vi "ziModGetSweeperHeader.vi"(8 "Error In":errorcluster, 10 "ModResults":T2, 11 "ModHandle In":T5 {"ModHandle" format="0x%08x"; "Conn" format="0x%08x"}) -> (0 "Error Out":errorcluster, 2 "SweeperHeader":T1[](array[typedef]), 3 "ModHandle Out":T5 {"ModHandle" format="0x%08x"; "Conn" format="0x%08x"})   [LabVIEW 2015, in "Zurich Instruments LabOne.lvlib"]
doc: "Use this vi to get Double Data from a ModResult returned from ziModGetNextNode.vi. It returns an array of Double Data."
uses:
  Zurich Instruments LabOne.lvlib
  ziTypeModSweeperHeader.ctl
  Zurich Instruments/LabOne/API/LabVIEW/Zurich Instruments LabOne/Private/ziLV64.framework
  Data/ziTypePollType.ctl
  ziTypeModHandle.ctl
  ziTypeModResults.ctl
  ziTypeModSWTriggerHeader.ctl
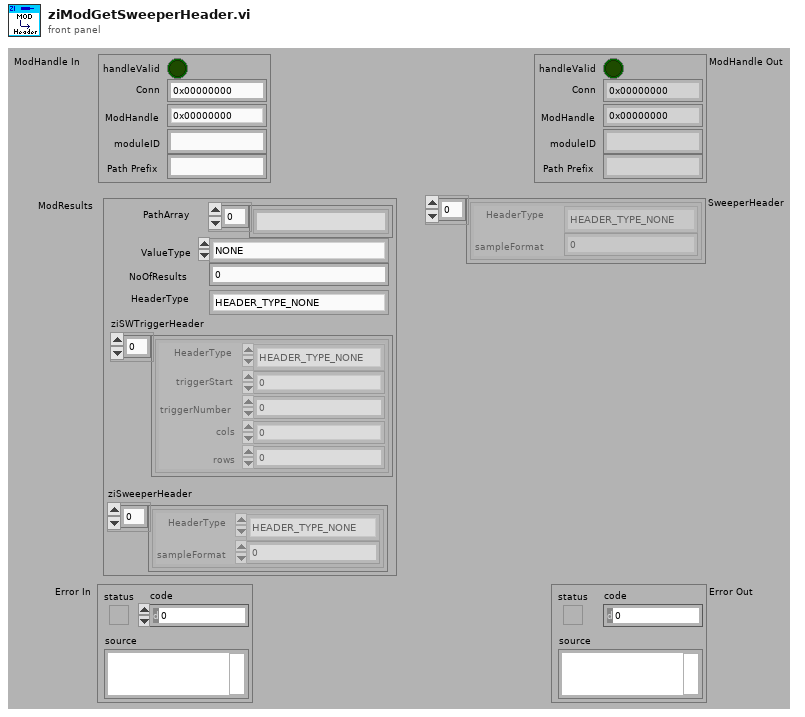
[diagram p1: front panel]
types:
  T1 = typedef "Zurich Instruments LabOne.lvlib/ziTypeModSweeperHeader.ctl" = cluster{"HeaderType":enum8{"HEADER_TYPE_NONE", "HEADER_TYPE_SWTRIGGER", "HEADER_TYPE_SWEEPER"}, "sampleFormat":u8}
  T2 = typedef "Zurich Instruments LabOne.lvlib/ziTypeModResults.ctl" = cluster{"PathArray":string[], "ValueType":T3, "NoOfResults":u64, "HeaderType":enum16{"HEADER_TYPE_NONE", "HEADER_TYPE_SWTRIGGER", "HEADER_TYPE_SWEEPER"}, "ziSWTriggerHeader":T4[], "ziSweeperHeader":T1[]}
  T3 = typedef "Zurich Instruments LabOne.lvlib/ziTypePollType.ctl" = enum16{"NONE", "DOUBLE_DATA", "INTEGER_DATA", "DEMOD_SAMPLE", "SCOPE_WAVE_HF2", "AUXIN_SAMPLE", "DIO_SAMPLE", "BYTE_ARRAY", "PWA_WAVE", "9", "10", "11", "12", "13", "14", "15", "TREE_CHANGE_DEPRI", "17", "ERROR", "19", "20", "21", "22", "23", "24", "25", "26", "27", "28", "29", "30", "31", "DOUBLE_DATA_TS", "INTEGER_DATA_TS", "34", "SCOPE_WAVE", "36", "37", "BYTE_ARRAY_TS", "39", "40", "41", "42", "43", "44", "45", "CNT_DATA", "47", "TREE_CHANGE", "49", "50", "51", "52", "53", "54", "55", "56", "57", "58", "59", "60", "61", "62", "63", "SWEEPER_DATA", "SPECTRUM_DATA", "ADVISOR_DATA", "67", "IMP_DATA"}
  T4 = typedef "Zurich Instruments LabOne.lvlib/ziTypeModSWTriggerHeader.ctl" = cluster{"HeaderType":enum8{"HEADER_TYPE_NONE", "HEADER_TYPE_SWTRIGGER", "HEADER_TYPE_SWEEPER"}, "triggerStart":u64, "triggerNumber":u64, "cols":u32, "rows":u32}
  T5 = typedef "Zurich Instruments LabOne.lvlib/ziTypeModHandle.ctl" = cluster{"handleValid":bool, "Conn":u64, "ModHandle":u64, "moduleID":string, "Path Prefix":string}
  T6 = enum16{"HEADER_TYPE_NONE", "HEADER_TYPE_SWTRIGGER", "HEADER_TYPE_SWEEPER"}
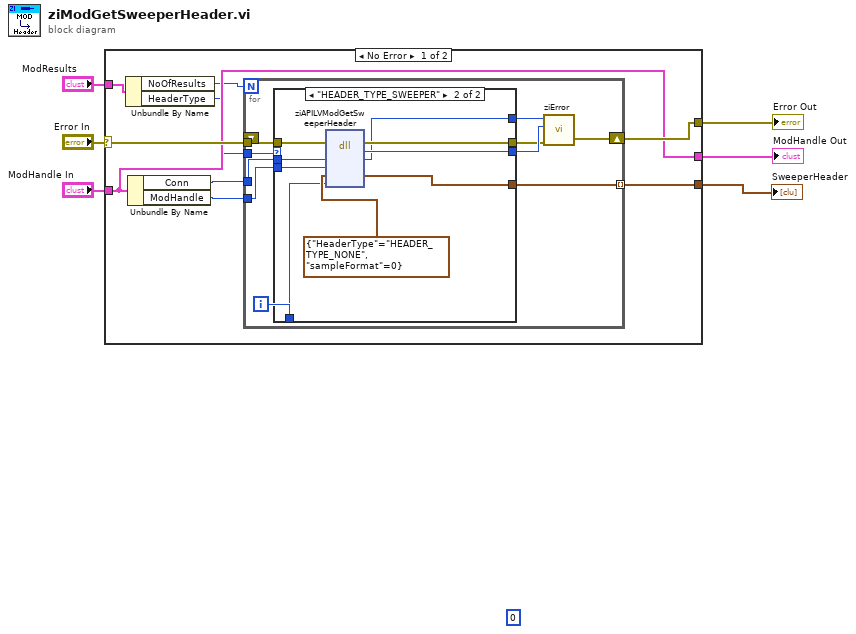
[diagram p0: block diagram]
diagram:
  (unwired) u64 0
  n1 = case shown="No Error" "Error In" {
    selector: "Error In" -> [w11 w37]
    tunnel: [w12 w37] -> w2
    tunnel: [w10 w38] -> w5
    tunnel: "ModHandle In" -> [w10 w38]
    tunnel: "ModResults" -> [w13 _]
    tunnel: [w9 _] -> w1
    frame No Error {
      n2 = Unbundle By Name(w13) -> ("NoOfResults"=w7:u64, "HeaderType"=w8:T6)
      n3 = Unbundle By Name(w10) -> ("Conn"=w15:u64, "ModHandle"=w14:u64)
      n4 = for {
        N: w7 -> [_]
        tunnel: w15 -> [w25]
        tunnel: w14 -> [w24]
        tunnel: w11 -> [w22]
        tunnel: [w21] -> w9 mode=indexing
        tunnel: w8 -> [w18]
        shift-right: [w23] -> w12
        shift-left: _ -> [_]
        i -> [w17]
        n5 = case shown="\"HEADER_TYPE_SWEEPER\"" w18 {
          tunnel: w25 -> [w26 w33]
          tunnel: w24 -> [_ w32]
          tunnel: [_ w31] -> w20
          tunnel: [w27 w36] -> w19
          tunnel: w22 -> [w27 w35]
          tunnel: [_ w30] -> w21
          tunnel: w17 -> [_ w29]
          tunnel: [w26 w28] -> w16
          frame "HEADER_TYPE_NONE", Default {
          }
          frame "HEADER_TYPE_SWEEPER" {
            n6 = dll-call lib="Users/arkady/Desktop/ado/github/resonant_ultrasound_arxiv/maglab ultrasound -- arkady --arxiv/Zurich Instruments/LabOne/API/LabVIEW/Zurich Instruments LabOne/Private/ziLV*.*" fn="ziAPILVModGetSweeperHeader"(error in=w35, "Conn"=w33, "ModHandle"=w32, "SWTriggerHeader"=T1 {"HeaderType"=enum."HEADER_TYPE_NONE", "sampleFormat"=0} ("ziModResults"), "chunk_idx"=w29) -> (error out=w36:errorcluster, "return type"=w31:u32, "Conn"=w28:u64, "SWTriggerHeader"=w30:T1)  [unwired: 4 in, 1 out]
          }
        }
        n7 = call "ziError.vi"("Conn"=w16, "ziErrorCode"=w20, "Error In"=w19) -> ("Error Out"=w23:errorcluster)  [unwired: 2 in, 1 out]
      }
    }
    frame Error {
    }
  }
  "Error Out" <- w2
  "ModHandle Out" <- w5
  "SweeperHeader" <- w1
